vi "Get Category.vi"(8 "error in (no error)":errorcluster, 11 "ThreePhasePLL editor node in":refnum<class "ThreePhasePLL editor node.lvclass">) -> (0 "error out":errorcluster, 2 "Category":string, 3 "ThreePhasePLL editor node out":refnum<class "ThreePhasePLL editor node.lvclass">)   [LabVIEW 2017, in "ThreePhasePLL editor node.lvclass"]
uses:
  ThreePhasePLL editor node.lvclass
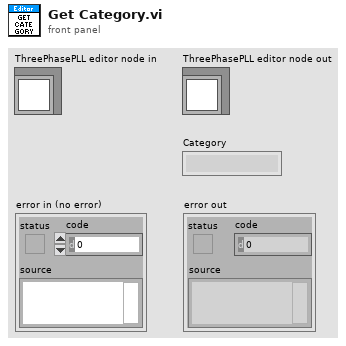
[diagram p1: front panel]
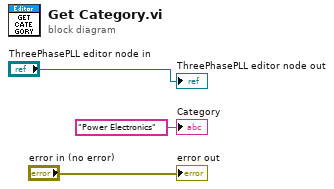
[diagram p0: block diagram]
diagram:
  "error out" <- "error in (no error)"
  "ThreePhasePLL editor node out" <- "ThreePhasePLL editor node in"
  "Category" <- "Power Electronics" ("Category")
